vi "PCO_ConvertSet.vi"(8 "error in (no error)":errorcluster {"code" format="%x"}, 10 "strConvert":T1, 11 "ph":u64) -> (0 "error out":errorcluster {"code" format="%x"}, 2 "ErrorMessage":i32 format="%x", 3 "ph out":u64)   [LabVIEW 2019, in "Convert.lvlib"]
doc: "int PCOCONVERT_API PCO_ConvertSet(HANDLE ph, PCO_Convert* pstrConvert);"
uses:
  Convert.lvlib
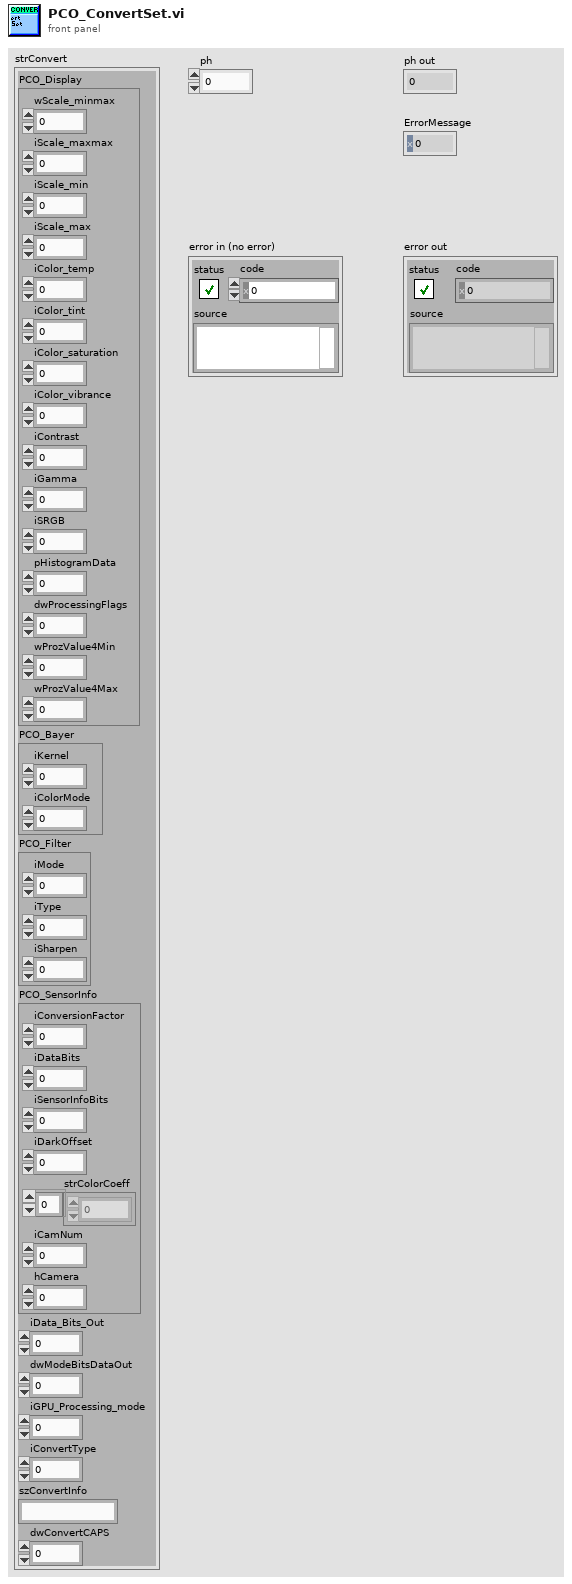
[diagram p1: front panel]
types:
  T1 = cluster{"PCO_Display":cluster{"wScale_minmax":u16, "iScale_maxmax":i32, "iScale_min":i32, "iScale_max":i32, "iColor_temp":i32, "iColor_tint":i32, "iColor_saturation":i32, "iColor_vibrance":i32, "iContrast":i32, "iGamma":i32, "iSRGB":i32, "pHistogramData":u64, "dwProcessingFlags":u32, "wProzValue4Min":u16, "wProzValue4Max":u16}, "PCO_Bayer":cluster{"iKernel":i32, "iColorMode":i32}, "PCO_Filter":cluster{"iMode":i32, "iType":i32, "iSharpen":i32}, "PCO_SensorInfo":cluster{"iConversionFactor":i32, "iDataBits":i32, "iSensorInfoBits":i32, "iDarkOffset":i32, "strColorCoeff":dbl[], "iCamNum":i32, "hCamera":u64}, "iData_Bits_Out":i32, "dwModeBitsDataOut":u32, "iGPU_Processing_mode":i32, "iConvertType":i32, "szConvertInfo":string, "dwConvertCAPS":u32}
  T2 = cluster{"wScale_minmax":u16, "iScale_maxmax":i32, "iScale_min":i32, "iScale_max":i32, "iColor_temp":i32, "iColor_tint":i32, "iColor_saturation":i32, "iColor_vibrance":i32, "iContrast":i32, "iGamma":i32, "iSRGB":i32, "pHistogramData":u64, "dwProcessingFlags":u32, "wProzValue4Min":u16, "wProzValue4Max":u16}
  T3 = cluster{"iMode":i32, "iType":i32, "iSharpen":i32}
  T4 = cluster{"iConversionFactor":i32, "iDataBits":i32, "iSensorInfoBits":i32, "iDarkOffset":i32, "strColorCoeff":dbl[], "iCamNum":i32, "hCamera":u64}
  T5 = cluster{"unsigned byte array[0]":u8, "unsigned byte array[1]":u8, "unsigned byte array[2]":u8, "unsigned byte array[3]":u8, "unsigned byte array[4]":u8, "unsigned byte array[5]":u8, "unsigned byte array[6]":u8, "unsigned byte array[7]":u8, "unsigned byte array[8]":u8, "unsigned byte array[9]":u8, "unsigned byte array[10]":u8, "unsigned byte array[11]":u8, "unsigned byte array[12]":u8, "unsigned byte array[13]":u8, "unsigned byte array[14]":u8, "unsigned byte array[15]":u8, "unsigned byte array[16]":u8, "unsigned byte array[17]":u8, "unsigned byte array[18]":u8, "unsigned byte array[19]":u8, "unsigned byte array[20]":u8, "unsigned byte array[21]":u8, "unsigned byte array[22]":u8, "unsigned byte array[23]":u8, "unsigned byte array[24]":u8, "unsigned byte array[25]":u8, "unsigned byte array[26]":u8, "unsigned byte array[27]":u8, "unsigned byte array[28]":u8, "unsigned byte array[29]":u8, "unsigned byte array[30]":u8, "unsigned byte array[31]":u8, "unsigned byte array[32]":u8, "unsigned byte array[33]":u8, "unsigned byte array[34]":u8, "unsigned byte array[35]":u8, "unsigned byte array[36]":u8, "unsigned byte array[37]":u8, "unsigned byte array[38]":u8, "unsigned byte array[39]":u8, "unsigned byte array[40]":u8, "unsigned byte array[41]":u8, "unsigned byte array[42]":u8, "unsigned byte array[43]":u8, "unsigned byte array[44]":u8, "unsigned byte array[45]":u8, "unsigned byte array[46]":u8, "unsigned byte array[47]":u8, "unsigned byte array[48]":u8, "unsigned byte array[49]":u8, "unsigned byte array[50]":u8, "unsigned byte array[51]":u8, "unsigned byte array[52]":u8, "unsigned byte array[53]":u8, "unsigned byte array[54]":u8, "unsigned byte array[55]":u8, "unsigned byte array[56]":u8, "unsigned byte array[57]":u8, "unsigned byte array[58]":u8, "unsigned byte array[59]":u8}
  T6 = cluster{"wSize":u16, "wScale_minmax":u16, "iScale_maxmax":i32, "iScale_min":i32, "iScale_max":i32, "iColor_temp":i32, "iColor_tint":i32, "iColor_saturation":i32, "iColor_vibrance":i32, "iContrast":i32, "iGamma":i32, "iSRGB":i32, "pHistogramData":u64, "dwDialogOpenFlags":u32, "dwProcessingFlags":u32, "wProzValue4Min":u16, "wProzValue4Max":u16, "dwzzDummy1":cluster{u32, u32, u32, u32, u32, u32, u32, u32, u32, u32, u32, u32, u32, u32, u32, u32, u32, u32, u32, u32, u32, u32, u32, u32, u32, u32, u32, u32, u32, u32, u32, u32, u32, u32, u32, u32, u32, u32, u32, u32, u32, u32, u32, u32, u32, u32, u32, u32, u32, u32}}
  T7 = cluster{"wSize":u16, "wScale_minmax":u16, "iScale_maxmax":i32, "iScale_min":i32, "iScale_max":i32, "iColor_temp":i32, "iColor_tint":i32, "iColor_saturation":i32, "iColor_vibrance":i32, "iContrast":i32, "iGamma":i32, "iSRGB":i32, "pHistogramData":u32, "dwDialogOpenFlags":u32, "dwProcessingFlags":u32, "wProzValue4Min":u16, "wProzValue4Max":u16, "dwzzDummy1":cluster{u32, u32, u32, u32, u32, u32, u32, u32, u32, u32, u32, u32, u32, u32, u32, u32, u32, u32, u32, u32, u32, u32, u32, u32, u32, u32, u32, u32, u32, u32, u32, u32, u32, u32, u32, u32, u32, u32, u32, u32, u32, u32, u32, u32, u32, u32, u32, u32, u32}}
  T8 = cluster{"wSize":u16, "wDummy":u16, "iKernel":i32, "iColorMode":i32, "dwzzDummy1":cluster{u32, u32, u32, u32, u32, u32, u32, u32, u32, u32, u32, u32, u32, u32, u32, u32, u32, u32, u32, u32, u32, u32, u32, u32, u32, u32, u32, u32, u32, u32, u32, u32, u32, u32, u32, u32, u32, u32, u32, u32, u32, u32, u32, u32, u32, u32, u32, u32, u32, u32, u32, u32, u32, u32, u32, u32, u32, u32, u32, u32, u32}}
  T9 = cluster{"wSize":u16, "wDummy":u16, "iMode":i32, "iType":i32, "iSharpen":i32, "dwzzDummy1":cluster{u32, u32, u32, u32, u32, u32, u32, u32, u32, u32, u32, u32, u32, u32, u32, u32, u32, u32, u32, u32, u32, u32, u32, u32, u32, u32, u32, u32, u32, u32, u32, u32, u32, u32, u32, u32, u32, u32, u32, u32, u32, u32, u32, u32, u32, u32, u32, u32, u32, u32, u32, u32, u32, u32, u32, u32, u32, u32, u32, u32}}
  T10 = cluster{"strColorCoeff[0]":dbl, "strColorCoeff[1]":dbl, "strColorCoeff[2]":dbl, "strColorCoeff[3]":dbl, "strColorCoeff[4]":dbl, "strColorCoeff[5]":dbl, "strColorCoeff[6]":dbl, "strColorCoeff[7]":dbl, "strColorCoeff[8]":dbl}
  T11 = cluster{"wSize":u16, "wDummy":u16, "iConversionFactor":i32, "iDataBits":i32, "iSensorInfoBits":i32, "iDarkOffset":i32, "dwzzDummy0":u32, "strColorCoeff":cluster{dbl, dbl, dbl, dbl, dbl, dbl, dbl, dbl, dbl}, "iCamNum":i32, "hCamera":u64, "dwzzDummy1":cluster{u32, u32, u32, u32, u32, u32, u32, u32, u32, u32, u32, u32, u32, u32, u32, u32, u32, u32, u32, u32, u32, u32, u32, u32, u32, u32, u32, u32, u32, u32, u32, u32, u32, u32, u32, u32, u32, u32, u32}}
  T12 = cluster{"wSize":u16, "wDummy":u16, "iConversionFactor":i32, "iDataBits":i32, "iSensorInfoBits":i32, "iDarkOffset":i32, "dwzzDummy0":u32, "strColorCoeff":cluster{dbl, dbl, dbl, dbl, dbl, dbl, dbl, dbl, dbl}, "iCamNum":i32, "hCamera":u32, "dwzzDummy1":cluster{u32, u32, u32, u32, u32, u32, u32, u32, u32, u32, u32, u32, u32, u32, u32, u32, u32, u32, u32, u32, u32, u32, u32, u32, u32, u32, u32, u32, u32, u32, u32, u32, u32, u32, u32, u32, u32, u32}}
  T13 = cluster{"wSize":u16, "wDummy":cluster{u16, u16, u16}, "PCO_DisplayRaw_x64":cluster{"wSize":u16, "wScale_minmax":u16, "iScale_maxmax":i32, "iScale_min":i32, "iScale_max":i32, "iColor_temp":i32, "iColor_tint":i32, "iColor_saturation":i32, "iColor_vibrance":i32, "iContrast":i32, "iGamma":i32, "iSRGB":i32, "pHistogramData":u64, "dwDialogOpenFlags":u32, "dwProcessingFlags":u32, "wProzValue4Min":u16, "wProzValue4Max":u16, "dwzzDummy1":cluster{u32, u32, u32, u32, u32, u32, u32, u32, u32, u32, u32, u32, u32, u32, u32, u32, u32, u32, u32, u32, u32, u32, u32, u32, u32, u32, u32, u32, u32, u32, u32, u32, u32, u32, u32, u32, u32, u32, u32, u32, u32, u32, u32, u32, u32, u32, u32, u32, u32, u32}}, "PCO_Bayer_Raw":cluster{"wSize":u16, "wDummy":u16, "iKernel":i32, "iColorMode":i32, "dwzzDummy1":cluster{u32, u32, u32, u32, u32, u32, u32, u32, u32, u32, u32, u32, u32, u32, u32, u32, u32, u32, u32, u32, u32, u32, u32, u32, u32, u32, u32, u32, u32, u32, u32, u32, u32, u32, u32, u32, u32, u32, u32, u32, u32, u32, u32, u32, u32, u32, u32, u32, u32, u32, u32, u32, u32, u32, u32, u32, u32, u32, u32, u32, u32}}, "PCO_Filter_Raw":cluster{"wSize":u16, "wDummy":u16, "iMode":i32, "iType":i32, "iSharpen":i32, "dwzzDummy1":cluster{u32, u32, u32, u32, u32, u32, u32, u32, u32, u32, u32, u32, u32, u32, u32, u32, u32, u32, u32, u32, u32, u32, u32, u32, u32, u32, u32, u32, u32, u32, u32, u32, u32, u32, u32, u32, u32, u32, u32, u32, u32, u32, u32, u32, u32, u32, u32, u32, u32, u32, u32, u32, u32, u32, u32, u32, u32, u32, u32, u32}}, "PCO_SensorInfo_Raw_x64":cluster{"wSize":u16, "wDummy":u16, "iConversionFactor":i32, "iDataBits":i32, "iSensorInfoBits":i32, "iDarkOffset":i32, "dwzzDummy0":u32, "strColorCoeff":cluster{dbl, dbl, dbl, dbl, dbl, dbl, dbl, dbl, dbl}, "iCamNum":i32, "hCamera":u64, "dwzzDummy1":cluster{u32, u32, u32, u32, u32, u32, u32, u32, u32, u32, u32, u32, u32, u32, u32, u32, u32, u32, u32, u32, u32, u32, u32, u32, u32, u32, u32, u32, u32, u32, u32, u32, u32, u32, u32, u32, u32, u32, u32}}, "iData_Bits_Out":i32, "dwModeBitsDataOut":u32, "iGPU_Processing_mode":i32, "iConvertType":i32, "szConvertInfo":cluster{u8, u8, u8, u8, u8, u8, u8, u8, u8, u8, u8, u8, u8, u8, u8, u8, u8, u8, u8, u8, u8, u8, u8, u8, u8, u8, u8, u8, u8, u8, u8, u8, u8, u8, u8, u8, u8, u8, u8, u8, u8, u8, u8, u8, u8, u8, u8, u8, u8, u8, u8, u8, u8, u8, u8, u8, u8, u8, u8, u8}, "dwConvertCAPS":u32, "dwzzDummy1":cluster{u32, u32, u32, u32, u32, u32, u32, u32, u32, u32, u32, u32, u32, u32, u32, u32, u32, u32, u32, u32, u32, u32, u32, u32, u32, u32, u32, u32, u32, u32, u32, u32, u32, u32, u32, u32, u32, u32, u32, u32, u32, u32}}
  T14 = cluster{"wSize":u16, "wDummy":cluster{u16, u16, u16}, "PCO_DisplayRaw_win32":cluster{"wSize":u16, "wScale_minmax":u16, "iScale_maxmax":i32, "iScale_min":i32, "iScale_max":i32, "iColor_temp":i32, "iColor_tint":i32, "iColor_saturation":i32, "iColor_vibrance":i32, "iContrast":i32, "iGamma":i32, "iSRGB":i32, "pHistogramData":u32, "dwDialogOpenFlags":u32, "dwProcessingFlags":u32, "wProzValue4Min":u16, "wProzValue4Max":u16, "dwzzDummy1":cluster{u32, u32, u32, u32, u32, u32, u32, u32, u32, u32, u32, u32, u32, u32, u32, u32, u32, u32, u32, u32, u32, u32, u32, u32, u32, u32, u32, u32, u32, u32, u32, u32, u32, u32, u32, u32, u32, u32, u32, u32, u32, u32, u32, u32, u32, u32, u32, u32, u32}}, "PCO_Bayer_Raw":cluster{"wSize":u16, "wDummy":u16, "iKernel":i32, "iColorMode":i32, "dwzzDummy1":cluster{u32, u32, u32, u32, u32, u32, u32, u32, u32, u32, u32, u32, u32, u32, u32, u32, u32, u32, u32, u32, u32, u32, u32, u32, u32, u32, u32, u32, u32, u32, u32, u32, u32, u32, u32, u32, u32, u32, u32, u32, u32, u32, u32, u32, u32, u32, u32, u32, u32, u32, u32, u32, u32, u32, u32, u32, u32, u32, u32, u32, u32}}, "PCO_Filter_Raw":cluster{"wSize":u16, "wDummy":u16, "iMode":i32, "iType":i32, "iSharpen":i32, "dwzzDummy1":cluster{u32, u32, u32, u32, u32, u32, u32, u32, u32, u32, u32, u32, u32, u32, u32, u32, u32, u32, u32, u32, u32, u32, u32, u32, u32, u32, u32, u32, u32, u32, u32, u32, u32, u32, u32, u32, u32, u32, u32, u32, u32, u32, u32, u32, u32, u32, u32, u32, u32, u32, u32, u32, u32, u32, u32, u32, u32, u32, u32, u32}}, "PCO_SensorInfo_Raw_win32":cluster{"wSize":u16, "wDummy":u16, "iConversionFactor":i32, "iDataBits":i32, "iSensorInfoBits":i32, "iDarkOffset":i32, "dwzzDummy0":u32, "strColorCoeff":cluster{dbl, dbl, dbl, dbl, dbl, dbl, dbl, dbl, dbl}, "iCamNum":i32, "hCamera":u32, "dwzzDummy1":cluster{u32, u32, u32, u32, u32, u32, u32, u32, u32, u32, u32, u32, u32, u32, u32, u32, u32, u32, u32, u32, u32, u32, u32, u32, u32, u32, u32, u32, u32, u32, u32, u32, u32, u32, u32, u32, u32, u32}}, "iData_Bits_Out":i32, "dwModeBitsDataOut":u32, "iGPU_Processing_mode":i32, "iConvertType":i32, "szConvertInfo":cluster{u8, u8, u8, u8, u8, u8, u8, u8, u8, u8, u8, u8, u8, u8, u8, u8, u8, u8, u8, u8, u8, u8, u8, u8, u8, u8, u8, u8, u8, u8, u8, u8, u8, u8, u8, u8, u8, u8, u8, u8, u8, u8, u8, u8, u8, u8, u8, u8, u8, u8, u8, u8, u8, u8, u8, u8, u8, u8, u8, u8}, "dwConvertCAPS":u32, "dwzzDummy1":cluster{u32, u32, u32, u32, u32, u32, u32, u32, u32, u32, u32, u32, u32, u32, u32, u32, u32, u32, u32, u32, u32, u32, u32, u32, u32, u32, u32, u32, u32, u32, u32, u32, u32, u32, u32, u32, u32, u32, u32, u32, u32, u32}}
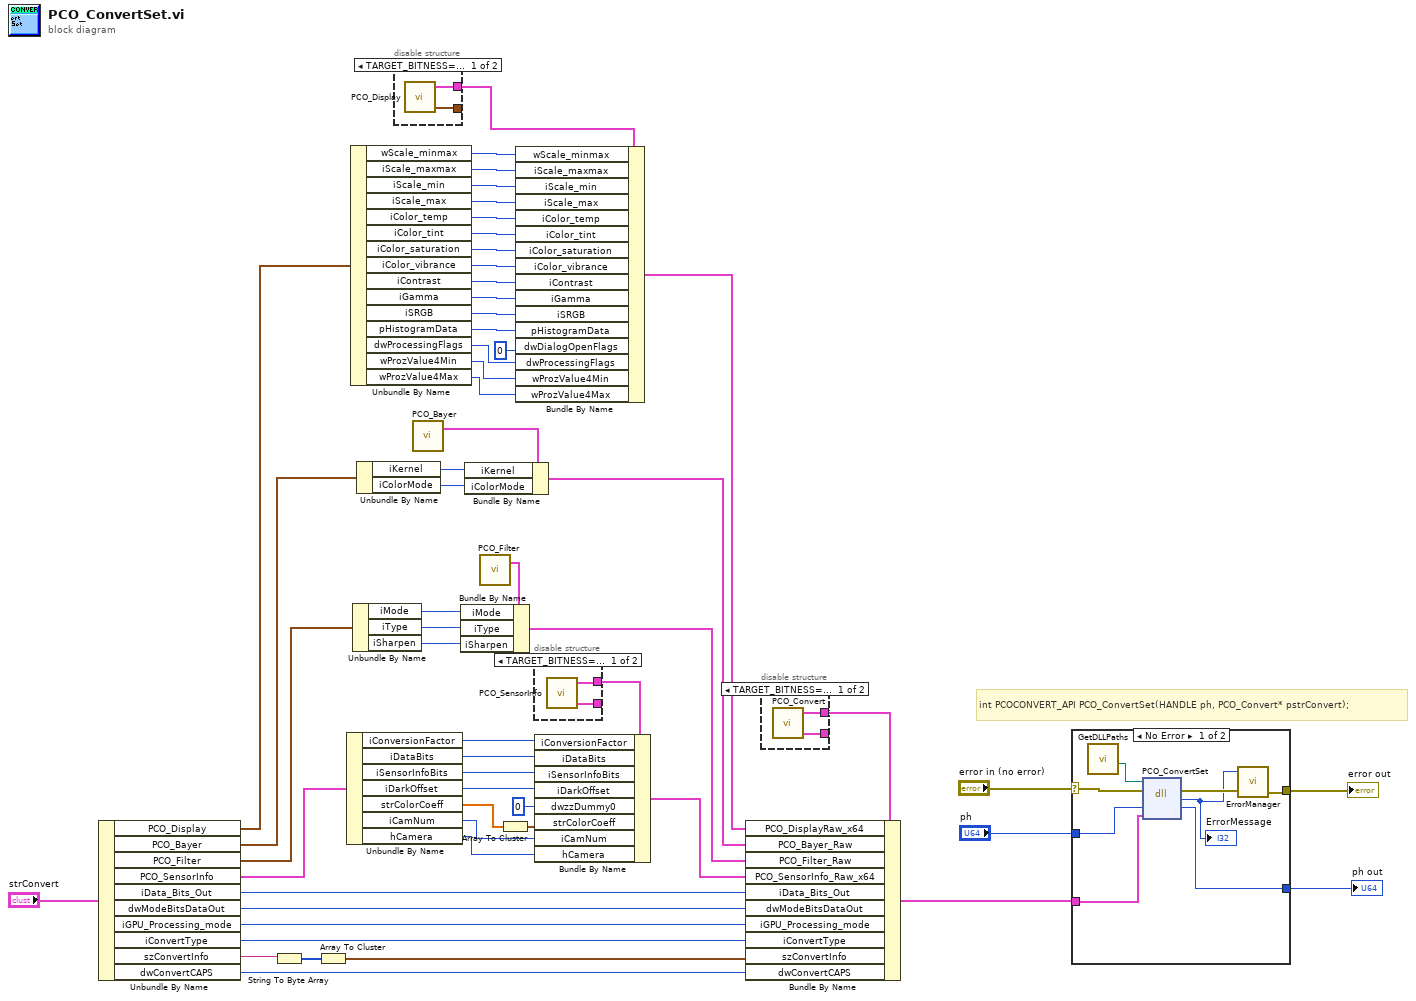
[diagram p0: block diagram]
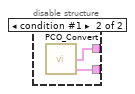
[diagram p2: hidden frame]
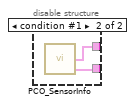
[diagram p3: hidden frame]
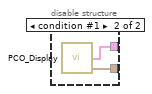
[diagram p4: hidden frame]
diagram:
  # "int PCOCONVERT_API PCO_ConvertSet(HANDLE ph, PCO_Convert* pstrConvert);"
  n1 = Unbundle By Name("strConvert") -> ("PCO_Display"=w52:T2, "PCO_Bayer"=w51:cluster{"iKernel":i32, "iColorMode":i32}, "PCO_Filter"=w50:T3, "PCO_SensorInfo"=w49:T4, "iData_Bits_Out"=w11:i32, "dwModeBitsDataOut"=w10:u32, "iGPU_Processing_mode"=w9:i32, "iConvertType"=w8:i32, "szConvertInfo"=w6:string, "dwConvertCAPS"=w7:u32)
  n2 = String To Byte Array(string=w6) -> (unsigned byte array=w5:u8[])
  n3 = Array To Cluster(array=w5) -> (cluster=w4:T5)
  n4 = Unbundle By Name(w49) -> ("iConversionFactor"=w31:i32, "iDataBits"=w30:i32, "iSensorInfoBits"=w29:i32, "iDarkOffset"=w28:i32, "strColorCoeff"=w27:dbl[], "iCamNum"=w25:i32, "hCamera"=w24:u64)
  n5 = Unbundle By Name(w52) -> ("wScale_minmax"=w47:u16, "iScale_maxmax"=w46:i32, "iScale_min"=w45:i32, "iScale_max"=w44:i32, "iColor_temp"=w43:i32, "iColor_tint"=w42:i32, "iColor_saturation"=w41:i32, "iColor_vibrance"=w40:i32, "iContrast"=w39:i32, "iGamma"=w38:i32, "iSRGB"=w37:i32, "pHistogramData"=w36:u64, "dwProcessingFlags"=w35:u32, "wProzValue4Min"=w34:u16, "wProzValue4Max"=w33:u16)
  n6 = Unbundle By Name(w50) -> ("iMode"=w22:i32, "iType"=w21:i32, "iSharpen"=w20:i32)
  n7 = Unbundle By Name(w51) -> ("iKernel"=w18:i32, "iColorMode"=w17:i32)
  n8 = disable-structure "Diagram Disable Structure" shown="TARGET_BITNESS==64, Default" {
    disable-tunnel: [w58 w61] -> _
    disable-tunnel: [w59 w60] -> w48
    frame condition #0 (active) {
      n9 = call "PCO_Display.vi"() -> ("PCO_DisplayRaw_x64"=w59:T6, "PCO_Display"=w58:T2)  [unwired: 4 in, 3 out]
    }
    frame condition #1 {
      n10 = call "PCO_Display.vi"() -> ("PCO_DisplayRaw_win32"=w60:T7, "PCO_Display"=w61:T2)  [unwired: 4 in, 3 out]
    }
  }
  n11 = call "PCO_Bayer.vi"() -> ("PCO_Bayer_Raw"=w19:T8)  [unwired: 4 in, 3 out]
  n12 = Bundle By Name(cluster=w19, "iKernel"=w18, "iColorMode"=w17) -> (w14:T8)
  n13 = call "PCO_Filter.vi"() -> ("PCO_Filter_Raw"=w23:T9)  [unwired: 4 in, 3 out]
  n14 = Bundle By Name(cluster=w23, "iMode"=w22, "iType"=w21, "iSharpen"=w20) -> (w13:T9)
  n15 = Array To Cluster(array=w27) -> (cluster=w26:T10)
  n16 = Bundle By Name(cluster=w48, "wScale_minmax"=w47, "iScale_maxmax"=w46, "iScale_min"=w45, "iScale_max"=w44, "iColor_temp"=w43, "iColor_tint"=w42, "iColor_saturation"=w41, "iColor_vibrance"=w40, "iContrast"=w39, "iGamma"=w38, "iSRGB"=w37, "pHistogramData"=w36, "dwDialogOpenFlags"=u32 0, "dwProcessingFlags"=w35, "wProzValue4Min"=w34, "wProzValue4Max"=w33) -> (w15:T6)
  n17 = disable-structure "Diagram Disable Structure" shown="TARGET_BITNESS==64, Default" {
    disable-tunnel: [w62 w65] -> _
    disable-tunnel: [w63 w64] -> w32
    frame condition #0 (active) {
      n18 = call "PCO_SensorInfo.vi"() -> ("PCO_SensorInfo_Raw_x64"=w63:T11, "PCO_SensorInfo"=w62:T4)  [unwired: 4 in, 3 out]
    }
    frame condition #1 {
      n19 = call "PCO_SensorInfo.vi"() -> ("PCO_SensorInfo_Raw_win32"=w64:T12, "PCO_SensorInfo"=w65:T4)  [unwired: 4 in, 3 out]
    }
  }
  n20 = Bundle By Name(cluster=w32, "iConversionFactor"=w31, "iDataBits"=w30, "iSensorInfoBits"=w29, "iDarkOffset"=w28, "dwzzDummy0"=u32 0, "strColorCoeff"=w26, "iCamNum"=w25, "hCamera"=w24) -> (w12:T11)
  n21 = disable-structure "Diagram Disable Structure" shown="TARGET_BITNESS==64, Default" {
    disable-tunnel: [w67 w69] -> _
    disable-tunnel: [w66 w68] -> w16
    frame condition #0 (active) {
      n22 = call "PCO_Convert.vi"() -> ("PCO_ConvertRaw_x64"=w66:T13, "PCO_Convert"=w67:T1)  [unwired: 4 in, 3 out]
    }
    frame condition #1 {
      n23 = call "PCO_Convert.vi"() -> ("PCO_ConvertRaw_win32"=w68:T14, "PCO_Convert"=w69:T1)  [unwired: 4 in, 3 out]
    }
  }
  n24 = Bundle By Name(cluster=w16, "PCO_DisplayRaw_x64"=w15, "PCO_Bayer_Raw"=w14, "PCO_Filter_Raw"=w13, "PCO_SensorInfo_Raw_x64"=w12, "iData_Bits_Out"=w11, "dwModeBitsDataOut"=w10, "iGPU_Processing_mode"=w9, "iConvertType"=w8, "szConvertInfo"=w4, "dwConvertCAPS"=w7) -> (w3:T13)
  n25 = case shown="No Error" "error in (no error)" {
    selector: "error in (no error)" -> [w74 w78]
    tunnel: "ph" -> [w77 w79]
    tunnel: [w76 w79] -> w56
    tunnel: w3 -> [w75 _]
    tunnel: [w72 w78] -> w55
    frame No Error {
      n26 = call "GetDLLPaths.vi"() -> ("PCO_Conv_Path"=w70:path)  [unwired: 8 in, 3 out]
      n27 = dll-call lib="?" fn="PCO_ConvertSet"(path in=w70, error in=w74, "ph"=w77, "pstrConvert"=w75) -> (error out=w73:errorcluster, "return type"=w71:i32, "ph"=w76:u64)  [unwired: 2 in, 1 out]
      "ErrorMessage" <- w71
      n28 = call "ErrorManager.vi"("error in (no error)"=w73, "error code"=w71) -> ("error out"=w72:errorcluster)  [unwired: 2 in, 1 out]
    }
    frame Error {
    }
  }
  "ph out" <- w56
  "error out" <- w55
